vi "Write.vi"(8 "Error In":errorcluster, 10 "Data":u8[](array[numeric]), 11 "SFTP File In":refnum<class "SFTP File.lvclass">) -> (0 "Error Out":errorcluster, 2 "Count":i64, 3 "SFTP File Out":refnum<class "SFTP File.lvclass">)   [LabVIEW 2018, in "Toolkit.lvlib" / "SFTP File.lvclass"]
uses:
  SFTP File.lvclass
  SFTP File.lvclass/SFTP File.ctl
  SFTP/SFTP.lvclass/SFTP.ctl
  Toolkit.lvlib
  SFTP/SFTP.lvclass
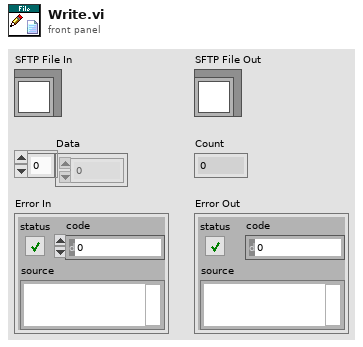
[diagram p1: front panel]
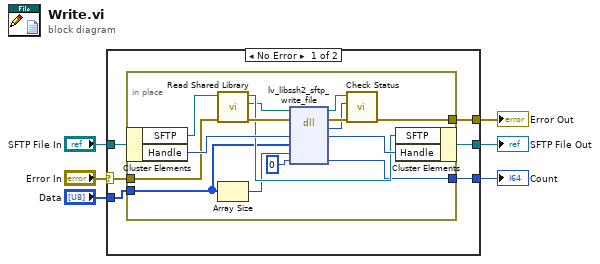
[diagram p0: block diagram]
diagram:
  n1 = case shown="No Error" "Error In" {
    selector: "Error In" -> [w11 w28]
    tunnel: "SFTP File In" -> [w12 w29]
    tunnel: [w10 w29] -> w3
    tunnel: [w9 w28] -> w4
    tunnel: "Data" -> [w8 _]
    tunnel: [w7 _] -> w1
    frame No Error {
      n2 = in-place {
        in-place-border: w11 -> [w26]
        in-place-border: [w21] -> w9
        in-place-border: w8 -> [w15]
        in-place-border: [w13] -> w7
        n3 = in-place-cluster #1(w12) -> ("SFTP"=w18:refnum<class "SFTP.lvclass">, "Handle"=w27:u64)
        n4 = call "Read Shared Library.vi"("Error In"=w26, "SFTP In"=w18) -> ("Erorr Out"=w19:errorcluster, "lv-libssh2 Shared Library"=w16:path, "SFTP Out"=w17:refnum<class "SFTP.lvclass">)  [unwired: 7 in]
        n5 = Array Size(array=w15) -> (size(s)=w14:i32)
        n6 = dll-call lib="libssh2lv.*" fn="lv_libssh2_sftp_write_file"(path in=w16, error in=w19, "handle"=w27, "buffer"=w15, "buffer_length"=w14, "write_count"=i64 0 ("read_count")) -> (path out=w23:path, error out=w24:errorcluster, "status"=w22:i32, "handle"=w25:u64, "write_count"=w13:i64)  [unwired: 3 in]
        n7 = call "Check Status.vi"("Error In"=w24, "Status"=w22, "lv-libssh2 Shared Library In"=w23) -> ("Error Out"=w21:errorcluster)  [unwired: 7 in, 1 out]
        n8 = in-place-cluster #1("SFTP"=w17, "Handle"=w25) -> (w10:refnum<class "SFTP File.lvclass">)
      }
    }
    frame Error {
    }
  }
  "Error Out" <- w4
  "SFTP File Out" <- w3
  "Count" <- w1
